vi "remote_sender.vi"(8 "error in":errorcluster, 11 "remote_queue":refnum<queue>) -> ()   [LabVIEW 2018]
uses:
  remote_mods.ctl
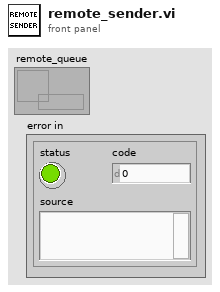
[diagram p1: front panel]
types:
  T1 = typedef "remote_mods.ctl" = enum16{"create", "send", "reconnect", "destroy"}
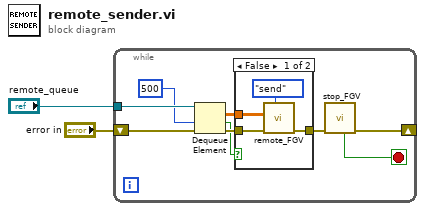
[diagram p0: block diagram]
diagram:
  n1 = while {
    tunnel: "remote_queue" -> [w11]
    shift-right: [w5] -> _
    shift-left: "error in" -> [w9]
    stop <- w4 stop-if-true
    n2 = Dequeue Element(queue=w11, timeout in ms (-1)=500, error in (no error)=w9) -> (element=w7:dbl[][], timed out?=w3:bool, error out=w8:errorcluster)  [unwired: 1 out]
    n3 = case shown="False" w3 {
      tunnel: w8 -> [w14 w16]
      tunnel: w7 -> [w13 _]
      tunnel: [w12 w16] -> w6
      frame False {
        n4 = call "remote_FGV.vi"("remote_mods"=remote_mods."send", "error in"=w14, "data"=w13) -> ("error out"=w12:errorcluster)  [unwired: 8 in]
      }
      frame True {
      }
    }
    n5 = call "stop_FGV.vi"("error in"=w6) -> ("error out"=w5:errorcluster, "parar?"=w4:bool)  [unwired: 9 in]
  }
